vi "LSMcontroller_v64_updatedwaveformhandling.vi"() -> ()   [LabVIEW 2015] (continued)
                                n2114 = property on="downright" class="Bool (strict)"("Value"=w5072) -> ()  [unwired: 2 in, 2 out]
                                }
                                }
                                }
                                }
                                }
                              }
                              n2115 = dll-call lib="phlib.dll" fn="_PH_GetCountRate@8" label="PH_GetCountRate"("devidx"=w5019, "channel"=1) -> (→"Ch1Rate":i32)  [unwired: 5 in, 2 out]
                              n2116 = local read "Stop"() -> (w5021:bool)
                              n2117 = local write "points recorded"(w5018) -> ()
                            }
                          }
                          frame #3 {
                            w5081 = FALSE ("Value (Signaling)")
                            n2118 = call "2pparameters.vi"("command"="get") -> ("params out"=w5075:T10)  [unwired: 1 in]
                            n2119 = Unbundle By Name(w5075) -> ("autoshutter"=w5076:bool)
                            n2120 = case shown="True" w5076 {
                              frame False {
                              }
                              frame True {
                                n2121 = call "shuttercontrol.vi"("command"="close") -> ()  [unwired: 1 in, 1 out]
                              }
                            }
                            n2122 = property on="Start" class="Bool (strict)"("Val(Sgnl)"=w5081) -> ()  [unwired: 2 in, 2 out]
                            n2123 = property on="Start" class="Bool (strict)"("Visible"=TRUE, "DisabledEnum"=T7."Enabled" ("Disabled")) -> ()  [unwired: 2 in, 2 out]
                            n2124 = property on="Stop" class="Bool (strict)"("Val(Sgnl)"=w5081) -> ()  [unwired: 2 in, 2 out]
                            n2125 = property on="Stop" class="Bool (strict)"("Visible"=FALSE, "DisabledEnum"=T7."Disabled" ("Disabled")) -> ()  [unwired: 2 in, 2 out]
                          }
                        }
                      }
                      frame Enabled {
                      }
                    }
                    n2126 = local write "64bit disabled"(TRUE ("64bit disabled")) -> ()
                  }
                }
              }
            }
          }
          event "avpp", "Angle ref", "xpixels ref", "Vx-min ref", "Vx-max ref", "ypixels ref", "Vy-min ref", "Vy-max ref", "ROI Type", "Sampling rate": Value Change {
            n2127 = event-data() -> ()  [unwired: 1 in, 6 out]
            n2128 = local read "avpp"() -> (w5100:i32)
            n2129 = local read "Angle ref"() -> (w5099:dbl)
            n2130 = local read "ROI Type"() -> (w5098:u16)
            n2131 = local read "xpixels ref"() -> (w5095:i32)
            n2132 = local read "Vx-min ref"() -> (w5094:dbl)
            n2133 = local read "Vx-max ref"() -> (w5093:dbl)
            n2134 = local read "ypixels ref"() -> (w5091:i32)
            n2135 = local read "Vy-min ref"() -> (w5092:dbl)
            n2136 = local read "Vy-max ref"() -> (w5088:dbl)
            n2137 = local read "Sampling rate"() -> (w5083:dbl)
            n2138 = local read "# of frames"() -> (w5087:i32)
            n2139 = local read "maxbufferAI"() -> (w5086:i32)
            n2140 = local read "Override AI buffer"() -> (w5084:bool)
            n2141 = call "2pparameters.vi"("command"="get") -> ("params out"=w5097:T10)  [unwired: 1 in]
            n2142 = Bundle By Name(cluster=w5097, "avpp"=w5100, "Angle Img"=w5099, "Xpixels Img"=w5095, "Vx-min Img"=w5094, "VX-max Img"=w5093, "Ypixels Img"=w5091, "Vy-min Img"=w5092, "Vy-max Img"=w5088, "srate"=w5083, "srate Img"=w5083, "measpoints"=w5087, "maxbufferAI"=w5086, "Drawing Mode"=w5098, "Vz-reset"=0.0, "AIoverride"=w5084) -> (w5089:T10)
            n2143 = call "2pparameters.vi"("Params in"=w5089, "command"="set") -> ()  [unwired: 1 out]
          }
          event "# of frames": Value Change {
            n2144 = event-data() -> ()  [unwired: 1 in, 6 out]
            n2145 = local read "Meastab"() -> (w5101:enum32{"X-Y Image", "Linescan", "Timetrace"})
            n2146 = case shown="\"X-Y Image\", Default" w5101 {
              frame "X-Y Image", Default {
                n2147 = local read "# of frames"() -> (w5102:i32)
                n2148 = call "2pparameters.vi"("command"="get") -> ("params out"=w5106:T10)  [unwired: 1 in]
                n2149 = Bundle By Name(cluster=w5106, "measpoints"=w5102) -> (w5103:T10)
                n2150 = call "2pparameters.vi"("Params in"=w5103, "command"="set") -> ()  [unwired: 1 out]
              }
              frame "Linescan" {
                n2151 = local read "srateAODOtt"() -> (w5116:dbl)
                n2152 = local read "# of frames"() -> (w5112:i32)
                n2153 = local read "refreshtime"() -> (w5118:dbl)
                n2154 = local read "bin"() -> (w5113:dbl)
                n2155 = call "tt_timeandsamples.vi"("bin"=w5113, "refreshtime"=w5118, "srateAODOtt"=w5116, "tot#ofsamples"=w5112) -> ("refreshrate"=w5115:dbl, "refreshbuffer"=w5114:i32, "timetracecycles"=w5111:i32)  [unwired: 5 in]
                n2156 = call "2pparameters.vi"("command"="get") -> ("params out"=w5108:T10)  [unwired: 1 in]
                n2157 = Bundle By Name(cluster=w5108, "measpoints"=w5112, "tt_cycles"=w5111, "refreshbuffer"=w5114, "refreshrate"=w5115) -> (w5110:T10)
                n2158 = Reciprocal(x=w5115) -> (1/x=w5117:dbl)
                n2159 = local write "refreshtime"(w5117) -> ()
                n2160 = call "2pparameters.vi"("Params in"=w5110, "command"="set") -> ()  [unwired: 1 out]
              }
              frame "Timetrace" {
                n2161 = local read "srateAODOtt"() -> (w5128:dbl)
                n2162 = local read "# of frames"() -> (w5124:i32)
                n2163 = local read "refreshtime"() -> (w5130:dbl)
                n2164 = local read "bin"() -> (w5125:dbl)
                n2165 = call "tt_timeandsamples.vi"("bin"=w5125, "refreshtime"=w5130, "srateAODOtt"=w5128, "tot#ofsamples"=w5124) -> ("refreshrate"=w5127:dbl, "refreshbuffer"=w5126:i32, "timetracecycles"=w5123:i32)  [unwired: 5 in]
                n2166 = call "2pparameters.vi"("command"="get") -> ("params out"=w5120:T10)  [unwired: 1 in]
                n2167 = Bundle By Name(cluster=w5120, "measpoints"=w5124, "tt_cycles"=w5123, "refreshbuffer"=w5126, "refreshrate"=w5127) -> (w5122:T10)
                n2168 = Reciprocal(x=w5127) -> (1/x=w5129:dbl)
                n2169 = local write "refreshtime"(w5129) -> ()
                n2170 = call "2pparameters.vi"("Params in"=w5122, "command"="set") -> ()  [unwired: 1 out]
              }
            }
          }
          event "srateAODOtt", "refreshtime", "Vx-ref", "Vy-ref", "Vx-min draw", "Vx-max draw", "Vy-min draw", "Vy-max draw", "bin": Value Change {
            n2171 = event-data() -> ()  [unwired: 1 in, 6 out]
            n2172 = local read "ypixels ref"() -> (w5162:i32)
            n2173 = local read "Vy-min draw"() -> (w5138:dbl)
            n2174 = local read "Vy-max draw"() -> (w5137:dbl)
            n2175 = local read "Vx-min draw"() -> (w5140:dbl)
            n2176 = local read "Vx-max draw"() -> (w5139:dbl)
            n2177 = local read "xpixels ref"() -> (w5136:i32)
            n2178 = local read "ROI Type"() -> (w5135:u16)
            n2179 = local read "Pel"() -> (w5134:dbl)
            n2180 = local read "srateAODOtt"() -> (w5144:dbl)
            n2181 = local read "# of frames"() -> (w5149:i32)
            n2182 = local read "refreshtime"() -> (w5142:dbl)
            n2183 = local read "bin"() -> (w5147:dbl)
            n2184 = local read "Override AI buffer"() -> (w5132:bool)
            n2185 = local read "finite samples"() -> (w5156:bool)
            n2186 = local read "srateAODOtt"() -> (w5131:dbl)
            n2187 = local read "srateAODOtt"() -> (w5150:dbl)
            n2188 = local read "continuous"() -> (w5155:bool)
            n2189 = local read "Angle ref"() -> (w5141:dbl)
            n2190 = local read "wavdet"() -> (w5157:bool)
            n2191 = local read "Vx-ref"() -> (w5152:dbl)
            n2192 = local read "Vy-ref"() -> (w5154:dbl)
            n2193 = local read "avpp"() -> (w5153:i32)
            n2194 = call "tt_timeandsamples.vi"("bin"=w5147, "refreshtime"=w5142, "srateAODOtt"=w5144, "tot#ofsamples"=w5149) -> ("refreshrate"=w5145:dbl, "refreshbuffer"=w5146:i32, "timetracecycles"=w5151:i32)  [unwired: 5 in]
            n2195 = local read "bin"() -> (w5148:dbl)
            n2196 = call "2pparameters.vi"("command"="get") -> ("params out"=w5160:T10)  [unwired: 1 in]
            n2197 = Bundle By Name(cluster=w5160, "Drawing Mode"=w5135, "measpoints"=w5149, "tt_cycles"=w5151, "refreshbuffer"=w5146, "refreshrate"=w5145, "Vx-ref"=w5152, "Vy-ref"=w5154, "srate"=w5131, "finite"=w5156, "cont"=w5155, "wavdet"=w5157, "avpp"=w5153, "srateAODO"=w5150, "bufferAI"=w5146, "bin"=w5148, "Angle Img"=w5141, "Vxminref"=w5140, "Vxmaxref"=w5139, "Vyminref"=w5138, "Vymaxref"=w5137, "Xpixels Img"=w5136, "Ypixels Img"=w5162, "Pel"=w5134, "Vz-reset"=0.0, "AIoverride"=w5132) -> (w5158:T10)
            n2198 = Reciprocal(x=w5145) -> (1/x=w5143:dbl)
            n2199 = local write "refreshtime"(w5143) -> ()
            n2200 = call "2pparameters.vi"("Params in"=w5158, "command"="set") -> ()  [unwired: 1 out]
          }
          event "Init": Value Change {
            # "Disabled for conversion to 64 bit"
            n2201 = event-data() -> ()  [unwired: 1 in, 6 out]
            n2202 = disable-structure shown="Disabled" {
              frame Disabled {
                n2203 = flat-sequence {
                  frame #0 {
                    n2204 = local read "Measurement"() -> (w5164:T4)
                    n2205 = case shown="\"Lifetime (scan)\", \"Lifetime (contour)\"" w5164 {
                      frame "X-Y-t movie", Default {
                      }
                      frame "Lifetime (point)" {
                        n2206 = stacked-sequence {
                          frame #0 {
                            n2207 = call "initialize.vi"("mode"=0) -> ()
                          }
                          frame #1 {
                            n2208 = call "calib.vi"() -> ()  [unwired: 1 in]
                          }
                        }
                      }
                      frame "Lifetime (scan)", "Lifetime (contour)" {
                        n2209 = stacked-sequence {
                          frame #0 {
                            n2210 = call "initialize.vi"("mode"=3) -> ()
                          }
                          frame #1 {
                            n2211 = call "calib.vi"() -> ()  [unwired: 1 in]
                          }
                        }
                      }
                    }
                  }
                  frame #1 {
                    n2212 = property on="Start" class="Bool (strict)"("Visible"=TRUE, "DisabledEnum"=T7."Enabled" ("Disabled")) -> ()  [unwired: 2 in, 2 out]
                    n2213 = property on="Init" class="Bool (strict)"("Visible"=FALSE, "DisabledEnum"=T7."Disabled and Grayed Out" ("Disabled"), "Value"=FALSE ("Init")) -> ()  [unwired: 2 in, 2 out]
                  }
                }
              }
              frame Enabled {
              }
            }
            n2214 = local write "64bit disabled"(TRUE ("64bit disabled")) -> ()
          }
          event "Measurement": Value Change {
            n2215 = event-data() -> ()  [unwired: 1 in, 5 out]
            n2216 = case shown="\"X-Y-t movie\"" "Measurement" {
              frame "X-Y-t movie" {
                w5174 = T7."Disabled" ("Disabled")
                w5173 = FALSE ("Visible")
                n2217 = call "2pparameters.vi"("command"="get") -> ("params out"=w5184:T10)  [unwired: 1 in]
                n2218 = local write "graphtab"(T5."image" ("graphtab")) -> ()
                n2219 = local write "Save tab"(enum32{"withsave", "withoutsave"}."withsave" ("Save tab")) -> ()
                n2220 = Bundle By Name(cluster=w5184, "type"="X-Y-t movie") -> (w5182:T10)
                n2221 = call "2pparameters.vi"("Params in"=w5182, "command"="set") -> ()  [unwired: 1 out]
                n2222 = property on="refreshtime" class="DigNum (strict)"("Visible"=FALSE, "DisabledEnum"=T7."Disabled and Grayed Out" ("Disabled")) -> ()  [unwired: 2 in, 2 out]
                n2223 = property on="ttt" class="Enum (strict)"("Visible"=FALSE) -> ()  [unwired: 2 in, 2 out]
                n2224 = property on="# of frames" class="DigNum (strict)"("DisabledEnum"=T7."Enabled" ("Disabled"), "Caption.Text"="# of frames") -> ()  [unwired: 2 in, 2 out]
                n2225 = property on="continuous" class="Bool (strict)"("Visible"=TRUE, "DisabledEnum"=T7."Enabled" ("Disabled")) -> ()  [unwired: 2 in, 2 out]
                n2226 = property on="finite samples" class="Bool (strict)"("Visible"=TRUE, "DisabledEnum"=T7."Enabled" ("Disabled")) -> ()  [unwired: 2 in, 2 out]
                n2227 = property on="avpp" class="DigNum (strict)"("Visible"=TRUE, "DisabledEnum"=T7."Enabled" ("Disabled")) -> ()  [unwired: 2 in, 2 out]
                n2228 = property on="srateAODOtt" class="DigNum (strict)"("Visible"=FALSE, "DisabledEnum"=T7."Disabled" ("Disabled")) -> ()  [unwired: 2 in, 2 out]
                n2229 = local write "save\ndata"(TRUE ("save\ndata")) -> ()
                n2230 = property on="finite samples" class="Bool (strict)"("Val(Sgnl)"=TRUE ("continuous for display")) -> ()  [unwired: 2 in, 2 out]
                n2231 = property on="continuous" class="Bool (strict)"("Value"=FALSE ("continuous for display")) -> ()  [unwired: 2 in, 2 out]
                n2232 = property on="Current Average" class="DigNum (strict)"("Visible"=TRUE, "DisabledEnum"=T7."Enabled" ("Disabled")) -> ()  [unwired: 2 in, 2 out]
                n2233 = property on="img_CH1" class="IntGraph (strict)"("ZScale.Maximum"=7.0 ("Z Scale.Range:Maximum")) -> ()  [unwired: 2 in, 2 out]
                n2234 = property on="Sampling rate" class="DigNum (strict)"("Visible"=TRUE, "DisabledEnum"=T7."Enabled" ("Disabled")) -> ()  [unwired: 2 in, 2 out]
                n2235 = property on="Pel" class="DigNum (strict)"("Visible"=w5173, "DisabledEnum"=w5174) -> ()  [unwired: 2 in, 2 out]
                n2236 = property on="bin" class="DigNum (strict)"("Visible"=w5173, "DisabledEnum"=w5174) -> ()  [unwired: 2 in, 2 out]
                "Meastab" <- enum32{"X-Y Image", "Linescan", "Timetrace"}."X-Y Image" ("Meastab")
                "Zscantab" <- enum32{"withzscan", "withoutzscan", "lifetime"}."withoutzscan" ("Zscantab")
              }
              frame "X-Y-Z stack" {
                w5206 = T7."Disabled" ("Disabled")
                w5205 = FALSE ("Visible")
                n2237 = call "2pparameters.vi"("command"="get") -> ("params out"=w5216:T10)  [unwired: 1 in]
                n2238 = call "2pparameters.vi"("command"="get") -> ("params out"=w5220:T10)  [unwired: 1 in]
                n2239 = Bundle By Name(cluster=w5216, "type"="X-Y-Z stack") -> (w5214:T10)
                n2240 = Unbundle By Name(w5220) -> ("motorref"=w5219:refnum<k7>)
                n2241 = call "2pparameters.vi"("Params in"=w5214, "command"="set") -> ()  [unwired: 1 out]
                n2242 = local write "Zscantab"(enum32{"withzscan", "withoutzscan", "lifetime"}."withzscan" ("Zscantab")) -> ()
                n2243 = local write "Meastab"(enum32{"X-Y Image", "Linescan", "Timetrace"}."X-Y Image" ("Meastab")) -> ()
                n2244 = invoke class="MG17Motor" method="GetPosition"(reference=w5219, "lChanID"=0, "pfPosition"=sgl 0.0) -> ("pfPosition"=w5231:sgl)  [unwired: 2 in, 4 out]
                n2245 = property on="refreshtime" class="DigNum (strict)"("Visible"=FALSE, "DisabledEnum"=T7."Disabled and Grayed Out" ("Disabled")) -> ()  [unwired: 2 in, 2 out]
                n2246 = property on="ttt" class="Enum (strict)"("Visible"=FALSE) -> ()  [unwired: 2 in, 2 out]
                n2247 = Multiply(x=w5231, y=1000.0) -> (x*y=w5230:dbl)
                n2248 = local write "Actual Z position"(w5230) -> ()
                n2249 = local write "Save tab"(enum32{"withsave", "withoutsave"}."withsave" ("Save tab")) -> ()
                n2250 = property on="finite samples" class="Bool (strict)"("Visible"=FALSE, "DisabledEnum"=T7."Disabled and Grayed Out" ("Disabled")) -> ()  [unwired: 2 in, 2 out]
                n2251 = property on="avpp" class="DigNum (strict)"("Visible"=TRUE, "DisabledEnum"=T7."Enabled" ("Disabled")) -> ()  [unwired: 2 in, 2 out]
                n2252 = property on="continuous" class="Bool (strict)"("Visible"=FALSE, "DisabledEnum"=T7."Disabled and Grayed Out" ("Disabled")) -> ()  [unwired: 2 in, 2 out]
                n2253 = property on="img_CH1" class="IntGraph (strict)"("ZScale.Maximum"=7.0 ("Z Scale.Range:Maximum")) -> ()  [unwired: 2 in, 2 out]
                n2254 = property on="srateAODOtt" class="DigNum (strict)"("Visible"=FALSE, "DisabledEnum"=T7."Disabled" ("Disabled")) -> ()  [unwired: 2 in, 2 out]
                n2255 = property on="Pel" class="DigNum (strict)"("Visible"=w5205, "DisabledEnum"=w5206) -> ()  [unwired: 2 in, 2 out]
                n2256 = property on="bin" class="DigNum (strict)"("Visible"=w5205, "DisabledEnum"=w5206) -> ()  [unwired: 2 in, 2 out]
                n2257 = property on="Current Average" class="DigNum (strict)"("Visible"=TRUE, "DisabledEnum"=T7."Enabled" ("Disabled")) -> ()  [unwired: 2 in, 2 out]
                n2258 = property on="# of frames" class="DigNum (strict)"("Caption.Text"="# of slices", "DisabledEnum"=T7."Disabled and Grayed Out" ("Disabled")) -> ()  [unwired: 2 in, 2 out]
                n2259 = local write "save\ndata"(TRUE ("save\ndata")) -> ()
                n2260 = property on="finite samples" class="Bool (strict)"("Val(Sgnl)"=TRUE ("continuous for display")) -> ()  [unwired: 2 in, 2 out]
                n2261 = property on="continuous" class="Bool (strict)"("Value"=FALSE ("continuous for display")) -> ()  [unwired: 2 in, 2 out]
                n2262 = property on="Sampling rate" class="DigNum (strict)"("Visible"=TRUE, "DisabledEnum"=T7."Enabled" ("Disabled")) -> ()  [unwired: 2 in, 2 out]
              }
              frame "X-Y-Z-t movie" {
                w5245 = T7."Disabled" ("Disabled")
                w5244 = FALSE ("Visible")
                n2263 = property on="# of frames" class="DigNum (strict)"("DisabledEnum"=T7."Enabled" ("Disabled")) -> ()  [unwired: 2 in, 2 out]
                n2264 = property on="Current Average" class="DigNum (strict)"("Visible"=TRUE, "DisabledEnum"=T7."Enabled" ("Disabled")) -> ()  [unwired: 2 in, 2 out]
                n2265 = property on="avpp" class="DigNum (strict)"("Visible"=TRUE, "DisabledEnum"=T7."Enabled" ("Disabled")) -> ()  [unwired: 2 in, 2 out]
                n2266 = local write "Save tab"(enum32{"withsave", "withoutsave"}."withsave" ("Save tab")) -> ()
                n2267 = local write "Zscantab"(enum32{"withzscan", "withoutzscan", "lifetime"}."withzscan" ("Zscantab")) -> ()
                n2268 = local write "Meastab"(enum32{"X-Y Image", "Linescan", "Timetrace"}."X-Y Image" ("Meastab")) -> ()
                n2269 = property on="refreshtime" class="DigNum (strict)"("Visible"=FALSE, "DisabledEnum"=T7."Disabled and Grayed Out" ("Disabled")) -> ()  [unwired: 2 in, 2 out]
                n2270 = property on="ttt" class="Enum (strict)"("Visible"=FALSE) -> ()  [unwired: 2 in, 2 out]
                n2271 = call "2pparameters.vi"("command"="get") -> ("params out"=w5255:T10)  [unwired: 1 in]
                n2272 = Bundle By Name(cluster=w5255, "type"="X-Y-Z-t movie") -> (w5253:T10)
                n2273 = property on="continuous" class="Bool (strict)"("Visible"=TRUE, "DisabledEnum"=T7."Enabled" ("Disabled")) -> ()  [unwired: 2 in, 2 out]
                n2274 = property on="finite samples" class="Bool (strict)"("Visible"=TRUE, "DisabledEnum"=T7."Enabled" ("Disabled")) -> ()  [unwired: 2 in, 2 out]
                n2275 = call "2pparameters.vi"("Params in"=w5253, "command"="set") -> ()  [unwired: 1 out]
                n2276 = property on="srateAODOtt" class="DigNum (strict)"("Visible"=FALSE, "DisabledEnum"=T7."Disabled" ("Disabled")) -> ()  [unwired: 2 in, 2 out]
                n2277 = local write "save\ndata"(TRUE ("save\ndata")) -> ()
                n2278 = property on="img_CH1" class="IntGraph (strict)"("ZScale.Maximum"=7.0 ("Z Scale.Range:Maximum")) -> ()  [unwired: 2 in, 2 out]
                n2279 = property on="continuous" class="Bool (strict)"("Value"=FALSE ("continuous for display")) -> ()  [unwired: 2 in, 2 out]
                n2280 = property on="finite samples" class="Bool (strict)"("Value"=TRUE ("continuous for display")) -> ()  [unwired: 2 in, 2 out]
                n2281 = property on="Sampling rate" class="DigNum (strict)"("Visible"=TRUE, "DisabledEnum"=T7."Enabled" ("Disabled")) -> ()  [unwired: 2 in, 2 out]
                n2282 = property on="Pel" class="DigNum (strict)"("Visible"=w5244, "DisabledEnum"=w5245) -> ()  [unwired: 2 in, 2 out]
                n2283 = property on="bin" class="DigNum (strict)"("Visible"=w5244, "DisabledEnum"=w5245) -> ()  [unwired: 2 in, 2 out]
              }
              frame "linescan" {
                w5275 = T7."Enabled" ("Disabled")
                w5274 = TRUE ("Visible")
                w5277 = T7."Enabled" ("Disabled")
                w5276 = TRUE ("Visible")
                n2284 = local write "Meastab"(enum32{"X-Y Image", "Linescan", "Timetrace"}."Linescan" ("Meastab")) -> ()
                n2285 = property on="Current Average" class="DigNum (strict)"("Visible"=TRUE, "DisabledEnum"=T7."Enabled" ("Disabled")) -> ()  [unwired: 2 in, 2 out]
                n2286 = local write "Save tab"(enum32{"withsave", "withoutsave"}."withsave" ("Save tab")) -> ()
                n2287 = local write "Zscantab"(enum32{"withzscan", "withoutzscan", "lifetime"}."withoutzscan" ("Zscantab")) -> ()
                n2288 = property on="refreshtime" class="DigNum (strict)"("Visible"=FALSE, "DisabledEnum"=T7."Disabled and Grayed Out" ("Disabled")) -> ()  [unwired: 2 in, 2 out]
                n2289 = property on="continuous" class="Bool (strict)"("Value"=FALSE ("continuous for display")) -> ()  [unwired: 2 in, 2 out]
                n2290 = property on="finite samples" class="Bool (strict)"("Value"=TRUE ("continuous for display")) -> ()  [unwired: 2 in, 2 out]
                n2291 = property on="ttt" class="Enum (strict)"("Visible"=FALSE) -> ()  [unwired: 2 in, 2 out]
                n2292 = local write "save\ndata"(TRUE ("save\ndata")) -> ()
                n2293 = call "2pparameters.vi"("command"="get") -> ("params out"=w5286:T10)  [unwired: 1 in]
                n2294 = Bundle By Name(cluster=w5286, "type"="linescan") -> (w5284:T10)
                n2295 = property on="# of frames" class="DigNum (strict)"("DisabledEnum"=T7."Enabled" ("Disabled"), "Caption.Text"="# of lines") -> ()  [unwired: 2 in, 2 out]
                n2296 = property on="continuous" class="Bool (strict)"("Visible"=TRUE, "DisabledEnum"=T7."Enabled" ("Disabled")) -> ()  [unwired: 2 in, 2 out]
                n2297 = property on="avpp" class="DigNum (strict)"("Visible"=TRUE, "DisabledEnum"=T7."Enabled" ("Disabled")) -> ()  [unwired: 2 in, 2 out]
                n2298 = property on="finite samples" class="Bool (strict)"("Visible"=TRUE, "DisabledEnum"=T7."Enabled" ("Disabled")) -> ()  [unwired: 2 in, 2 out]
                n2299 = property on="srateAODOtt" class="DigNum (strict)"("Visible"=TRUE, "DisabledEnum"=T7."Enabled" ("Disabled")) -> ()  [unwired: 2 in, 2 out]
                n2300 = call "2pparameters.vi"("Params in"=w5284, "command"="set") -> ()  [unwired: 1 out]
                n2301 = property on="Pel" class="DigNum (strict)"("Visible"=w5276, "DisabledEnum"=w5277) -> ()  [unwired: 2 in, 2 out]
                n2302 = property on="bin" class="DigNum (strict)"("Visible"=w5276, "DisabledEnum"=w5277) -> ()  [unwired: 2 in, 2 out]
                n2303 = property on="Sampling rate" class="DigNum (strict)"("Visible"=FALSE, "DisabledEnum"=T7."Disabled" ("Disabled")) -> ()  [unwired: 2 in, 2 out]
                n2304 = property on="Pel" class="DigNum (strict)"("Visible"=w5274, "DisabledEnum"=w5275) -> ()  [unwired: 2 in, 2 out]
                n2305 = property on="bin" class="DigNum (strict)"("Visible"=w5274, "DisabledEnum"=w5275) -> ()  [unwired: 2 in, 2 out]
              }
              frame "Timetrace" {
                w5307 = T7."Enabled" ("Disabled")
                w5306 = TRUE ("Visible")
                n2306 = call "2pparameters.vi"("command"="get") -> ("params out"=w5312:T10)  [unwired: 1 in]
                n2307 = local write "Meastab"(enum32{"X-Y Image", "Linescan", "Timetrace"}."Timetrace" ("Meastab")) -> ()
                n2308 = Unbundle By Name(w5312) -> ("Angle draw"=w5314:dbl)
                n2309 = local write "Zscantab"(enum32{"withzscan", "withoutzscan", "lifetime"}."withoutzscan" ("Zscantab")) -> ()
                n2310 = property on="# of frames" class="DigNum (strict)"("DisabledEnum"=T7."Enabled" ("Disabled"), "Caption.Text"="# of samples") -> ()  [unwired: 2 in, 2 out]
                n2311 = property on="refreshtime" class="DigNum (strict)"("Visible"=TRUE, "DisabledEnum"=T7."Enabled" ("Disabled")) -> ()  [unwired: 2 in, 2 out]
                n2312 = property on="avpp" class="DigNum (strict)"("Visible"=FALSE, "DisabledEnum"=T7."Disabled and Grayed Out" ("Disabled")) -> ()  [unwired: 2 in, 2 out]
                n2313 = property on="Current Average" class="DigNum (strict)"("Visible"=FALSE, "DisabledEnum"=T7."Disabled and Grayed Out" ("Disabled")) -> ()  [unwired: 2 in, 2 out]
                n2314 = local write "Angle drawing"(w5314) -> ()
                n2315 = property on="ttt" class="Enum (strict)"("Visible"=TRUE) -> ()  [unwired: 2 in, 2 out]
                n2316 = property on="continuous" class="Bool (strict)"("Visible"=TRUE, "DisabledEnum"=T7."Enabled" ("Disabled")) -> ()  [unwired: 2 in, 2 out]
                n2317 = property on="finite samples" class="Bool (strict)"("Visible"=TRUE, "DisabledEnum"=T7."Enabled" ("Disabled")) -> ()  [unwired: 2 in, 2 out]
                n2318 = local write "save\ndata"(TRUE ("save\ndata")) -> ()
                n2319 = property on="finite samples" class="Bool (strict)"("Val(Sgnl)"=TRUE ("continuous for display")) -> ()  [unwired: 2 in, 2 out]
                n2320 = property on="continuous" class="Bool (strict)"("Value"=FALSE ("continuous for display")) -> ()  [unwired: 2 in, 2 out]
                n2321 = local write "Save tab"(enum32{"withsave", "withoutsave"}."withsave" ("Save tab")) -> ()
                n2322 = property on="srateAODOtt" class="DigNum (strict)"("Visible"=TRUE, "DisabledEnum"=T7."Enabled" ("Disabled")) -> ()  [unwired: 2 in, 2 out]
                n2323 = call "2pparameters.vi"("command"="get") -> ("params out"=w5319:T10)  [unwired: 1 in]
                n2324 = Bundle By Name(cluster=w5319, "type"="Timetrace") -> (w5317:T10)
                n2325 = property on="Sampling rate" class="DigNum (strict)"("Visible"=FALSE, "DisabledEnum"=T7."Disabled" ("Disabled")) -> ()  [unwired: 2 in, 2 out]
                n2326 = property on="Pel" class="DigNum (strict)"("Visible"=w5306, "DisabledEnum"=w5307) -> ()  [unwired: 2 in, 2 out]
                n2327 = property on="bin" class="DigNum (strict)"("Visible"=w5306, "DisabledEnum"=w5307) -> ()  [unwired: 2 in, 2 out]
                n2328 = call "2pparameters.vi"("Params in"=w5317, "command"="set") -> ()  [unwired: 1 out]
              }
              frame "Lifetime (point)" {
                w5340 = T7."Enabled" ("Disabled")
                w5339 = TRUE ("Visible")
                n2329 = property on="Pel" class="DigNum (strict)"("Visible"=w5339, "DisabledEnum"=w5340) -> ()  [unwired: 2 in, 2 out]
                n2330 = property on="bin" class="DigNum (strict)"("Visible"=w5339, "DisabledEnum"=w5340) -> ()  [unwired: 2 in, 2 out]
                n2331 = property on="ttt" class="Enum (strict)"("Visible"=FALSE) -> ()  [unwired: 2 in, 2 out]
                n2332 = local write "Zscantab"(enum32{"withzscan", "withoutzscan", "lifetime"}."lifetime" ("Zscantab")) -> ()
                n2333 = local write "graphtab"(T5."Lifetime" ("graphtab")) -> ()
                n2334 = local write "Meastab"(enum32{"X-Y Image", "Linescan", "Timetrace"}."Timetrace" ("Meastab")) -> ()
                n2335 = call "lifetimeparameters.vi"("command"="get") -> ("Params out"=w5347:T19)  [unwired: 1 in]
                n2336 = Unbundle By Name(w5347) -> ("initialized"=w5348:bool)
                n2337 = property on="srateAODOtt" class="DigNum (strict)"("Visible"=TRUE, "DisabledEnum"=T7."Enabled" ("Disabled")) -> ()  [unwired: 2 in, 2 out]
                n2338 = case shown="False" w5348 {
                  frame False {
                    n2339 = property on="Init" class="Bool (strict)"("Visible"=TRUE, "DisabledEnum"=T7."Enabled" ("Disabled")) -> ()  [unwired: 2 in, 2 out]
                    n2340 = property on="Start" class="Bool (strict)"("Visible"=FALSE, "DisabledEnum"=T7."Disabled and Grayed Out" ("Disabled")) -> ()  [unwired: 2 in, 2 out]
                  }
                  frame True {
                  }
                }
                n2341 = property on="Sampling rate" class="DigNum (strict)"("Visible"=FALSE, "DisabledEnum"=T7."Disabled" ("Disabled")) -> ()  [unwired: 2 in, 2 out]
              }
              frame "Lifetime (scan)" {
                w5357 = T7."Disabled" ("Disabled")
                w5356 = FALSE ("Visible")
                n2342 = call "lifetimeparameters.vi"("command"="get") -> ("Params out"=w5369:T19)  [unwired: 1 in]
                n2343 = local write "graphtab"(T5."image" ("graphtab")) -> ()
                n2344 = local write "Save tab"(enum32{"withsave", "withoutsave"}."withsave" ("Save tab")) -> ()
                n2345 = local write "Meastab"(enum32{"X-Y Image", "Linescan", "Timetrace"}."X-Y Image" ("Meastab")) -> ()
                n2346 = local write "Zscantab"(enum32{"withzscan", "withoutzscan", "lifetime"}."lifetime" ("Zscantab")) -> ()
                n2347 = Unbundle By Name(w5369) -> ("initialized"=w5368:bool)
                n2348 = property on="ttt" class="Enum (strict)"("Visible"=FALSE) -> ()  [unwired: 2 in, 2 out]
                n2349 = property on="refreshtime" class="DigNum (strict)"("Visible"=FALSE, "DisabledEnum"=T7."Disabled and Grayed Out" ("Disabled")) -> ()  [unwired: 2 in, 2 out]
                n2350 = property on="Pel" class="DigNum (strict)"("Visible"=w5356, "DisabledEnum"=w5357) -> ()  [unwired: 2 in, 2 out]
                n2351 = property on="bin" class="DigNum (strict)"("Visible"=w5356, "DisabledEnum"=w5357) -> ()  [unwired: 2 in, 2 out]
                n2352 = property on="save data" class="Bool (strict)"("Visible"=TRUE, "DisabledEnum"=T7."Enabled" ("Disabled"), "Value"=TRUE ("Visible")) -> ()  [unwired: 2 in, 2 out]
                n2353 = case shown="False" w5368 {
                  frame False {
                    n2354 = property on="Init" class="Bool (strict)"("Visible"=TRUE, "DisabledEnum"=T7."Enabled" ("Disabled")) -> ()  [unwired: 2 in, 2 out]
                    n2355 = property on="Start" class="Bool (strict)"("Visible"=FALSE, "DisabledEnum"=T7."Disabled and Grayed Out" ("Disabled")) -> ()  [unwired: 2 in, 2 out]
                  }
                  frame True {
                  }
                }
                n2356 = call "2pparameters.vi"("command"="get") -> ("params out"=w5374:T10)  [unwired: 1 in]
                n2357 = property on="continuous" class="Bool (strict)"("Visible"=TRUE, "DisabledEnum"=T7."Disabled and Grayed Out" ("Disabled")) -> ()  [unwired: 2 in, 2 out]
                n2358 = property on="finite samples" class="Bool (strict)"("Visible"=TRUE, "DisabledEnum"=T7."Enabled" ("Disabled")) -> ()  [unwired: 2 in, 2 out]
                n2359 = Bundle By Name(cluster=w5374, "type"="Lifetime (scan)") -> (w5372:T10)
                n2360 = call "2pparameters.vi"("Params in"=w5372, "command"="set") -> ()  [unwired: 1 out]
                n2361 = property on="finite samples" class="Bool (strict)"("Val(Sgnl)"=TRUE ("continuous for display")) -> ()  [unwired: 2 in, 2 out]
                n2362 = property on="continuous" class="Bool (strict)"("Value"=FALSE ("continuous for display")) -> ()  [unwired: 2 in, 2 out]
                n2363 = property on="srateAODOtt" class="DigNum (strict)"("Visible"=FALSE, "DisabledEnum"=T7."Disabled" ("Disabled")) -> ()  [unwired: 2 in, 2 out]
                n2364 = property on="# of frames" class="DigNum (strict)"("DisabledEnum"=T7."Enabled" ("Disabled"), "Caption.Text"="# of frames") -> ()  [unwired: 2 in, 2 out]
                n2365 = property on="img_CH1" class="IntGraph (strict)"("ZScale.Maximum"=12.5 ("Z Scale.Range:Maximum")) -> ()  [unwired: 2 in, 2 out]
                n2366 = property on="Current Average" class="DigNum (strict)"("Visible"=TRUE, "DisabledEnum"=T7."Enabled" ("Disabled")) -> ()  [unwired: 2 in, 2 out]
                n2367 = property on="Sampling rate" class="DigNum (strict)"("Visible"=TRUE, "DisabledEnum"=T7."Enabled" ("Disabled")) -> ()  [unwired: 2 in, 2 out]
                n2368 = property on="avpp" class="DigNum (strict)"("Visible"=TRUE, "DisabledEnum"=T7."Enabled" ("Disabled")) -> ()  [unwired: 2 in, 2 out]
              }
              frame "Lifetime (contour)" {
                w5398 = T7."Enabled" ("Disabled")
                w5397 = TRUE ("Visible")
                n2369 = call "2pparameters.vi"("command"="get") -> ("params out"=w5405:T10)  [unwired: 1 in]
                n2370 = property on="# of frames" class="DigNum (strict)"("DisabledEnum"=T7."Enabled" ("Disabled"), "Caption.Text"="# of samples") -> ()  [unwired: 2 in, 2 out]
                n2371 = property on="refreshtime" class="DigNum (strict)"("Visible"=TRUE, "DisabledEnum"=T7."Enabled" ("Disabled")) -> ()  [unwired: 2 in, 2 out]
                n2372 = Unbundle By Name(w5405) -> ("Angle draw"=w5407:dbl)
                n2373 = property on="avpp" class="DigNum (strict)"("Visible"=FALSE, "DisabledEnum"=T7."Disabled and Grayed Out" ("Disabled")) -> ()  [unwired: 2 in, 2 out]
                n2374 = property on="Current Average" class="DigNum (strict)"("Visible"=FALSE, "DisabledEnum"=T7."Disabled and Grayed Out" ("Disabled")) -> ()  [unwired: 2 in, 2 out]
                n2375 = local write "Angle drawing"(w5407) -> ()
                n2376 = local write "Save tab"(enum32{"withsave", "withoutsave"}."withsave" ("Save tab")) -> ()
                n2377 = local write "Zscantab"(enum32{"withzscan", "withoutzscan", "lifetime"}."lifetime" ("Zscantab")) -> ()
                n2378 = local write "graphtab"(T5."Lifetime" ("graphtab")) -> ()
                n2379 = local write "Meastab"(enum32{"X-Y Image", "Linescan", "Timetrace"}."Timetrace" ("Meastab")) -> ()
                n2380 = property on="ttt" class="Enum (strict)"("Visible"=TRUE) -> ()  [unwired: 2 in, 2 out]
                n2381 = call "lifetimeparameters.vi"("command"="get") -> ("Params out"=w5429:T19)  [unwired: 1 in]
                n2382 = property on="finite samples" class="Bool (strict)"("Val(Sgnl)"=TRUE ("continuous for display")) -> ()  [unwired: 2 in, 2 out]
                n2383 = local write "save\ndata"(TRUE ("save\ndata")) -> ()
                n2384 = Unbundle By Name(w5429) -> ("initialized"=w5430:bool)
                n2385 = property on="continuous" class="Bool (strict)"("Visible"=TRUE, "DisabledEnum"=T7."Enabled" ("Disabled")) -> ()  [unwired: 2 in, 2 out]
                n2386 = property on="finite samples" class="Bool (strict)"("Visible"=TRUE, "DisabledEnum"=T7."Enabled" ("Disabled")) -> ()  [unwired: 2 in, 2 out]
                n2387 = property on="Pel" class="DigNum (strict)"("Visible"=w5397, "DisabledEnum"=w5398) -> ()  [unwired: 2 in, 2 out]
                n2388 = property on="bin" class="DigNum (strict)"("Visible"=w5397, "DisabledEnum"=w5398) -> ()  [unwired: 2 in, 2 out]
                n2389 = property on="continuous" class="Bool (strict)"("Value"=FALSE ("continuous for display")) -> ()  [unwired: 2 in, 2 out]
                n2390 = case shown="False" w5430 {
                  frame False {
                    n2391 = property on="Init" class="Bool (strict)"("Visible"=TRUE, "DisabledEnum"=T7."Enabled" ("Disabled")) -> ()  [unwired: 2 in, 2 out]
                    n2392 = property on="Start" class="Bool (strict)"("Visible"=FALSE, "DisabledEnum"=T7."Disabled and Grayed Out" ("Disabled")) -> ()  [unwired: 2 in, 2 out]
                  }
                  frame True {
                  }
                }
                n2393 = property on="srateAODOtt" class="DigNum (strict)"("Visible"=TRUE, "DisabledEnum"=T7."Enabled" ("Disabled")) -> ()  [unwired: 2 in, 2 out]
                n2394 = call "2pparameters.vi"("command"="get") -> ("params out"=w5409:T10)  [unwired: 1 in]
                n2395 = Bundle By Name(cluster=w5409, "type"="Timetrace") -> (w5403:T10)
                n2396 = call "2pparameters.vi"("Params in"=w5403, "command"="set") -> ()  [unwired: 1 out]
                n2397 = property on="Sampling rate" class="DigNum (strict)"("Visible"=FALSE, "DisabledEnum"=T7."Disabled" ("Disabled")) -> ()  [unwired: 2 in, 2 out]
              }
            }
          }
          event "Laserpower \n(%)": Value Change {
            n2398 = event-data() -> ("OldVal"=w5438:dbl, "NewVal"=w5439:dbl)  [unwired: 1 in, 4 out]
            n2399 = Not Equal?(x=w5438, y=w5439) -> (x != y?=w5440:bool)
            n2400 = case shown="True" w5440 {
              tunnel: w5439 -> [_ w5442]
              frame False {
              }
              frame True {
                n2401 = local read "wavelength(nm)"() -> (w5443:dbl)
                n2402 = call "configuration.vi"("command"="get") -> ("config out"=w5447:T11)  [unwired: 2 in, 1 out]
                n2403 = call "pockelscellcalibration.vi"("l"=w5443, "T"=w5442) -> ("Vout"=w5441:dbl)
                n2404 = Unbundle By Name(w5447) -> ("Vto2P"=w5446:i32, "AOlines"=w5445:tag[])
                n2405 = property on="lpow" class="DigNum (strict)"("Value"=w5442) -> ()  [unwired: 2 in, 2 out]
                n2406 = local write "Vpockels"(w5441) -> ()
                n2407 = Index Array(array=w5445, index=w5446) -> (element=w5444:tag)
                n2408 = call-poly <vilib>:"DAQmx Create Virtual Channel.vi"("physical channels"=w5444) -> ("task out"=w5450:refnum<k21>, "error out"=w5449:errorcluster)  [unwired: 13 in]
                n2409 = call-poly <vilib>:"DAQmx Write.vi"("task/channels in"=w5450, "data"=w5441, "error in"=w5449) -> ("task out"=w5451:refnum<k21>, "error out"=w5452:errorcluster)  [unwired: 10 in, 1 out]
                n2410 = call <vilib>:"DAQmx Start Task.vi"("task/channels in"=w5451, "error in"=w5452) -> ("task out"=w5453:refnum<k21>, "error out"=w5454:errorcluster)  [unwired: 12 in]
                n2411 = call <vilib>:"DAQmx Stop Task.vi"("task/channels in"=w5453, "error in"=w5454) -> ("task out"=w5455:refnum<k21>, "error out"=w5456:errorcluster)  [unwired: 12 in]
                n2412 = call <vilib>:"DAQmx Clear Task.vi"("task in"=w5455, "error in"=w5456) -> ()  [unwired: 13 in, 1 out]
              }
            }
          }
          event "lpow": Value Change {
            n2413 = event-data() -> ("OldVal"=w5457:dbl, "NewVal"=w5458:dbl)  [unwired: 1 in, 4 out]
            n2414 = Not Equal?(x=w5457, y=w5458) -> (x != y?=w5459:bool)
            n2415 = case shown="True" w5459 {
              tunnel: w5458 -> [_ w5462]
              frame False {
              }
              frame True {
                n2416 = local read "wavelength(nm)"() -> (w5461:dbl)
                n2417 = call "pockelscellcalibration.vi"("l"=w5461, "T"=w5462) -> ("Vout"=w5460:dbl)
                n2418 = call "configuration.vi"("command"="get") -> ("config out"=w5466:T11)  [unwired: 2 in, 1 out]
                n2419 = Unbundle By Name(w5466) -> ("Vto2P"=w5465:i32, "AOlines"=w5464:tag[])
                n2420 = local write "Vpockels"(w5460) -> ()
                n2421 = property on="Laserpower \n(%)" class="Slide (strict)"("Value"=w5462) -> ()  [unwired: 2 in, 2 out]
                n2422 = Index Array(array=w5464, index=w5465) -> (element=w5463:tag)
                n2423 = call-poly <vilib>:"DAQmx Create Virtual Channel.vi"("physical channels"=w5463) -> ("task out"=w5469:refnum<k21>, "error out"=w5468:errorcluster)  [unwired: 13 in]
                n2424 = call-poly <vilib>:"DAQmx Write.vi"("task/channels in"=w5469, "data"=w5460, "error in"=w5468) -> ("task out"=w5470:refnum<k21>, "error out"=w5471:errorcluster)  [unwired: 10 in, 1 out]
                n2425 = call <vilib>:"DAQmx Start Task.vi"("task/channels in"=w5470, "error in"=w5471) -> ("task out"=w5472:refnum<k21>, "error out"=w5473:errorcluster)  [unwired: 12 in]
                n2426 = call <vilib>:"DAQmx Stop Task.vi"("task/channels in"=w5472, "error in"=w5473) -> ("task out"=w5474:refnum<k21>, "error out"=w5475:errorcluster)  [unwired: 12 in]
                n2427 = call <vilib>:"DAQmx Clear Task.vi"("task in"=w5474, "error in"=w5475) -> ()  [unwired: 13 in, 1 out]
              }
            }
          }
          event "sealtest": Value Change {
            n2428 = event-data() -> ()  [unwired: 1 in, 6 out]
            n2429 = case shown="True" "sealtest" {
              frame False {
              }
              frame True {
                n2430 = stacked-sequence {
                  seq-local: [w5477 _ _ _ _ _] -> [_ w5510 _ w5562 _ _]
                  frame #0 {
                    n2431 = stacked-sequence {
                      tunnel: [_ w5489 _] -> w5477
                      frame #0 {
                        n2432 = call "2pparameters.vi"("command"="get") -> ("params out"=w5482:T10)  [unwired: 1 in]
                        n2433 = Unbundle By Name(w5482) -> ("autoshutter"=w5483:bool)
                        n2434 = local read "OCchecked?"() -> (w5480:bool)
                        n2435 = call "sealtestwfparams.vi"("command"="set") -> ()  [unwired: 6 in, 1 out]
                        n2436 = case shown="False" w5480 {
                          frame False {
                            n2437 = One Button Dialog(message="Is the OC gain correct?", button name ("OK")="ok") -> (true=w5484:bool)
                            n2438 = local write "OCchecked?"(w5484) -> ()
                          }
                          frame True {
                          }
                        }
                        n2439 = case shown="True" w5483 {
                          frame False {
                          }
                          frame True {
                            n2440 = call "shuttercontrol.vi"("command"="close") -> ()  [unwired: 1 in, 1 out]
                          }
                        }
                        n2441 = call "allAI-temp.vi"("command"=enum16{"get", "set", "clear", "append"}."clear") -> ()  [unwired: 3 in, 2 out]
                      }
                      frame #1 {
                        n2442 = call "sealtestwfparams.vi"("command"="get") -> ("Params out"=w5495:T22)  [unwired: 6 in]
                        n2443 = Unbundle By Name(w5495) -> ("AO parameters"=w5493:T23)
                        n2444 = Index Array(array=w5493, index=0) -> (element=w5492:T24)
                        n2445 = call "generateRampedSquareWave_fromAOparameters.vi"("AO params"=w5492) -> ("Waveform"=w5488:waveform(dbl), "wflength"=w5489:i32)
                        n2446 = Build Array(w5488) -> (w5491:waveform(dbl)[])
                        n2447 = call "waveformssealtestbuffer.vi"("AO wf in"=w5491, "command"="set") -> ()  [unwired: 1 out]
                      }
                      frame #2 {
                        n2448 = local read "Vholding (mV)"() -> (w5498:sgl)
                        n2449 = local read "Current Clamp"() -> (w5504:bool)
                        n2450 = local read "Voltage Clamp"() -> (w5503:bool)
                        n2451 = local read "OCgain"() -> (w5499:sgl)
                        n2452 = local read "CC_ICgain"() -> (w5502:dbl)
                        n2453 = local read "holdon"() -> (w5497:bool)
                        n2454 = call "patchparameters.vi"("command"="get") -> ("Params out"=w5506:T13)  [unwired: 1 in]
                        n2455 = Bundle By Name(cluster=w5506, "VC"=w5503, "CC"=w5504, "CC_icg (pA/mv)"=w5502, "VC_icg (mV/mV)"=10.0, "OCG (mV/pA)"=w5499, "OVG (mV/mV)"=0.1, "Vhold (mV)"=w5498, "holdon"=w5497) -> (w5505:T13)
                        n2456 = call "patchparameters.vi"("Params in"=w5505, "command"="set") -> ()  [unwired: 1 out]
                      }
                    }
                  }
                  frame #1 {
                    w5509 = 2
                    n2457 = call "patchparameters.vi"("command"="get") -> ("Params out"=w5517:T13)  [unwired: 1 in]
                    n2458 = Unbundle By Name(w5517) -> ("holdon"=w5516:bool, "Vhold (mV)"=w5515:sgl, "CC_icg (pA/mv)"=w5523:sgl, "CC"=w5521:bool, "VC_icg (mV/mV)"=w5522:sgl)
                    n2459 = Select(t=w5523, s=w5521, f=w5522) -> (s? t:f=w5524:sgl)
                    n2460 = To Single Precision Float(number=0.001 ("y")) -> (single precision float=w5525:sgl)
                    n2461 = Compound Arithmetic op=MULTIPLY(w5515, w5524, w5525) -> (w5519:sgl)
                    n2462 = case shown="False" w5516 {
                      tunnel: w5519 -> [_ w5537]
                      tunnel: [0.0 w5537] -> w5512
                      frame False {
                      }
                      frame True {
                      }
                    }
                    n2463 = Greater Than 0?(x=w5509) -> (x > 0?=w5511:bool)
                    n2464 = case shown="True" w5511 {
                      tunnel: w5510 -> [_ w5526]
                      tunnel: w5509 -> [_ w5529]
                      frame False {
                      }
                      frame True {
                        n2465 = Initialize Array(sgl 0.0 ("element"), w5529, w5526) -> (w5527:sgl[][])
                        n2466 = call "allAI-temp.vi"("array in"=w5527, "command"=enum16{"get", "set", "clear", "append"}."set") -> ()  [unwired: 2 in, 2 out]
                      }
                    }
                    n2467 = flat-sequence {
                      tunnel: w5510 -> [w5533]
                      tunnel: w5510 -> [w5532]
                      tunnel: [w5532] -> w5514
                      tunnel: [w5531] -> w5513
                      tunnel: w5512 -> [w5531]
                      tunnel: w5514 -> [w5535]
                      tunnel: w5513 -> [w5534]
                      frame #0 {
                        n2468 = call "prepAI_sealtest.vi"("samples per channel"=w5533) -> ()  [unwired: 2 in]
                      }
                      frame #1 {
                        n2469 = call "prepAO_sealtest.vi"("Vhold"=w5534, "samples per channel"=w5535) -> ()  [unwired: 1 in]
                      }
                    }
                  }
                  frame #2 {
                    n2470 = stacked-sequence {
                      frame #0 {
                        n2471 = call "tempconfigAO.vi"("command"="get") -> ("Temp Config out"=w5541:T25)  [unwired: 1 in]
                        n2472 = Unbundle By Name(w5541) -> ("AO"=w5542:refnum<k21>[], "E_AO"=w5543:errorcluster[])
                        n2473 = for {
                          tunnel: w5542 -> [w5551] mode=indexing
                          tunnel: w5543 -> [w5550] mode=indexing
                          tunnel: [w5549] -> w5545 mode=indexing
                          tunnel: [w5548] -> w5546 mode=indexing
                          n2474 = call <vilib>:"DAQmx Start Task.vi"("task/channels in"=w5551, "error in"=w5550) -> ("task out"=w5549:refnum<k21>, "error out"=w5548:errorcluster)  [unwired: 12 in]
                        }
                        n2475 = call "tempconfigAO.vi"("command"="get") -> ("Temp Config out"=w5544:T25)  [unwired: 1 in]
                        n2476 = Bundle By Name(cluster=w5544, "AO"=w5545, "E_AO"=w5546) -> (w5547:T25)
                        n2477 = call "tempconfigAO.vi"("Temp Config in"=w5547, "command"="set") -> ()  [unwired: 1 out]
                      }
                      frame #1 {
                        n2478 = call "tempconfigAI.vi"("command"="get") -> ("Temp Config out"=w5553:T26)  [unwired: 1 in]
                        n2479 = Unbundle By Name(w5553) -> ("AI"=w5558:refnum<k21>, "E_AI"=w5559:errorcluster)
                        n2480 = call <vilib>:"DAQmx Start Task.vi"("task/channels in"=w5558, "error in"=w5559) -> ("task out"=w5560:refnum<k21>, "error out"=w5561:errorcluster)  [unwired: 12 in]
                        n2481 = call "tempconfigAI.vi"("command"="get") -> ("Temp Config out"=w5555:T26)  [unwired: 1 in]
                        n2482 = Bundle By Name(cluster=w5555, "AI"=w5560, "E_AI"=w5561) -> (w5557:T26)
                        n2483 = call "tempconfigAI.vi"("Temp Config in"=w5557, "command"="set") -> ()  [unwired: 1 out]
                      }
                    }
                  }
                  frame #3 {
                    n2484 = while {
                      tunnel: w5562 -> [w5563]
                      stop <- w5564 stop-if-true
                      n2485 = local read "sealtest"() -> (w5567:bool)
                      n2486 = Not(x=w5567) -> (.not. x?=w5566:bool)
                      n2487 = case shown="False" w5566 {
                        tunnel: w5563 -> [w5568 _]
                        frame False {
                          n2488 = stacked-sequence {
                            seq-local: [_ _ _ w5607 _ _] -> [_ _ _ _ w5663 _]
                            seq-local: [w5569 _ _ _ _ _] -> [_ w5578 _ w5600 w5652 w5683]
                            tunnel: w5568 -> [_ _ w5586 _ w5651 _]
                            frame #0 {
                              n2489 = call "patchparameters.vi"("command"="get") -> ("Params out"=w5576:T13)  [unwired: 1 in]
                              n2490 = local read "Vholding (mV)"() -> (w5573:sgl)
                              n2491 = Unbundle By Name(w5576) -> ("Vhold (mV)"=w5572:sgl, "holdon"=w5575:bool)
                              n2492 = local read "holdon"() -> (w5574:bool)
                              n2493 = Not Equal?(x=w5573, y=w5572) -> (x != y?=w5571:bool)
                              n2494 = Not Equal?(x=w5575, y=w5574) -> (x != y?=w5570:bool)
                              n2495 = Or(x=w5571, y=w5570) -> (x .or. y?=w5569:bool)
                            }
                            frame #1 {
                              n2496 = case shown="True" w5578 {
                                frame False {
                                }
                                frame True {
                                n2497 = local read "Vholding (mV)"() -> (w5581:sgl)
                                n2498 = local read "holdon"() -> (w5579:bool)
                                n2499 = call "patchparameters.vi"("command"="get") -> ("Params out"=w5582:T13)  [unwired: 1 in]
                                n2500 = Bundle By Name(cluster=w5582, "Vhold (mV)"=w5581, "holdon"=w5579) -> (w5580:T13)
                                n2501 = call "patchparameters.vi"("Params in"=w5580, "command"="set") -> ()  [unwired: 1 out]
                                }
                              }
                            }
                            frame #2 {
                              n2502 = call "tempconfigAI.vi"("command"="get") -> ("Temp Config out"=w5596:T26)  [unwired: 1 in]
                              n2503 = Unbundle By Name(w5596) -> ("AI"=w5595:refnum<k21>, "E_AI"=w5594:errorcluster)
                              n2504 = call-poly <vilib>:"DAQmx Read.vi"("task/channels in"=w5595, "number of samples per channel"=w5586, "timeout"=10.0, "error in"=w5594) -> ("task out"=w5590:refnum<k21>, "data"=w5587:i16[][], "error out"=w5599:errorcluster)  [unwired: 9 in]
                              n2505 = call "tempconfigAI.vi"("command"="get") -> ("Temp Config out"=w5591:T26)  [unwired: 1 in]
                              n2506 = Bundle By Name(cluster=w5591, "AI"=w5590, "E_AI"=w5599) -> (w5598:T26)
                              n2507 = To Single Precision Float(number=w5587) -> (single precision float=w5589:sgl[][])
                              n2508 = call "tempconfigAI.vi"("Temp Config in"=w5598, "command"="set") -> ()  [unwired: 1 out]
                              n2509 = call "allAI-temp.vi"("array in"=w5589, "command"=enum16{"get", "set", "clear", "append"}."set") -> ()  [unwired: 2 in, 2 out]
                            }
                            frame #3 {
                              n2510 = case shown="True" w5600 {
                                frame False {
                                }
                                frame True {
                                n2511 = call "tempconfigAO.vi"("command"="get") -> ("Temp Config out"=w5640:T25)  [unwired: 1 in]
                                n2512 = Unbundle By Name(w5640) -> ("AO"=w5639:refnum<k21>[], "E_AO"=w5638:errorcluster[])
                                n2513 = call "tempconfigAI.vi"("command"="get") -> ("Temp Config out"=w5627:T26)  [unwired: 1 in]
                                n2514 = Unbundle By Name(w5627) -> ("AI"=w5628:refnum<k21>, "E_AI"=w5629:errorcluster)
                                n2515 = for {
                                tunnel: w5639 -> [w5644] mode=indexing
                                tunnel: w5638 -> [w5643] mode=indexing
                                tunnel: [w5642] -> w5634 mode=indexing
                                n2516 = call <vilib>:"DAQmx Stop Task.vi"("task/channels in"=w5644, "error in"=w5643) -> ("task out"=w5645:refnum<k21>, "error out"=w5646:errorcluster)  [unwired: 12 in]
                                n2517 = call <vilib>:"DAQmx Clear Task.vi"("task in"=w5645, "error in"=w5646) -> ("error out"=w5642:errorcluster)  [unwired: 13 in]
                                }
                                n2518 = call <vilib>:"DAQmx Stop Task.vi"("task/channels in"=w5628, "error in"=w5629) -> ("task out"=w5625:refnum<k21>, "error out"=w5624:errorcluster)  [unwired: 12 in]
                                n2519 = call <vilib>:"DAQmx Clear Task.vi"("task in"=w5625, "error in"=w5624) -> ("error out"=w5623:errorcluster)  [unwired: 13 in]
                                n2520 = call "tempconfigAO.vi"("command"="get") -> ("Temp Config out"=w5635:T25)  [unwired: 1 in]
                                n2521 = Bundle By Name(cluster=w5635, "E_AO"=w5634) -> (w5633:T25)
                                n2522 = call "tempconfigAI.vi"("command"="get") -> ("Temp Config out"=w5631:T26)  [unwired: 1 in]
                                n2523 = Bundle By Name(cluster=w5631, "E_AI"=w5623) -> (w5622:T26)
                                n2524 = call "tempconfigAO.vi"("Temp Config in"=w5633, "command"="set") -> ()  [unwired: 1 out]
                                n2525 = call "tempconfigAI.vi"("Temp Config in"=w5622, "command"="set") -> ()  [unwired: 1 out]
                                }
                              }
                              n2526 = call "allAI-temp.vi"("command"=enum16{"get", "set", "clear", "append"}."get") -> ("array out"=w5604:sgl[][])  [unwired: 3 in, 1 out]
                              n2527 = call "tempconfigAI.vi"("command"="get") -> ("Temp Config out"=w5617:T26)  [unwired: 1 in]
                              n2528 = call "tempconfigAI.vi"("command"="get") -> ("Temp Config out"=w5619:T26)  [unwired: 1 in]
                              n2529 = Unbundle By Name(w5617) -> ("header"=w5615:dbl[])
                              n2530 = Unbundle By Name(w5619) -> ("header"=w5621:dbl[])
                              n2531 = Index Array(array=w5604, index (row) #1=1 ("index (row)"), index (row) #2=0 ("index (row)")) -> (element #1=w5602:sgl[], element #2=w5601:sgl[])  [unwired: 2 in]
                              n2532 = local read "OCgain"() -> (w5609:sgl)
                              n2533 = call "Unscaledtoscaled.vi"("Unscaled Data"=w5602, "Header Information"=w5615) -> ("Array"=w5614:sgl[])  [unwired: 1 in]
                              n2534 = call "Unscaledtoscaled.vi"("Unscaled Data"=w5601, "Header Information"=w5621) -> ("Array"=w5618:sgl[])  [unwired: 1 in]
                              n2535 = Multiply(x=w5614, y=0.1) -> (x*y=w5611:dbl[])
                              n2536 = Divide(x=w5618, y=w5609) -> (x/y=w5610:sgl[])
                              n2537 = Build Array(w5611, w5610) -> (w5613:dbl[][])
                              n2538 = Multiply(x=w5613, y=1000.0) -> (x*y=w5607:dbl[][])
                              "Patch readout" <- w5607
                            }
                            frame #4 {
                              n2539 = case shown="True" w5652 {
                                tunnel: w5651 -> [_ w5664]
                                frame False {
                                }
                                frame True {
                                n2540 = call "patchparameters.vi"("command"="get") -> ("Params out"=w5668:T13)  [unwired: 1 in]
                                n2541 = Unbundle By Name(w5668) -> ("holdon"=w5667:bool, "Vhold (mV)"=w5666:sgl, "CC_icg (pA/mv)"=w5674:sgl, "CC"=w5672:bool, "VC_icg (mV/mV)"=w5673:sgl)
                                n2542 = Select(t=w5674, s=w5672, f=w5673) -> (s? t:f=w5675:sgl)
                                n2543 = To Single Precision Float(number=0.001 ("y")) -> (single precision float=w5676:sgl)
                                n2544 = Compound Arithmetic op=MULTIPLY(w5666, w5675, w5676) -> (w5670:sgl)
                                n2545 = case shown="True" w5667 {
                                tunnel: w5670 -> [_ w5681]
                                tunnel: [0.0 w5681] -> w5665
                                frame False {
                                }
                                frame True {
                                }
                                }
                                n2546 = flat-sequence {
                                tunnel: w5664 -> [w5677]
                                tunnel: w5665 -> [w5679]
                                tunnel: w5664 -> [w5678]
                                frame #0 {
                                n2547 = call "prepAI_sealtest.vi"("samples per channel"=w5677) -> ()  [unwired: 2 in]
                                }
                                frame #1 {
                                n2548 = call "prepAO_sealtest.vi"("Vhold"=w5679, "samples per channel"=w5678) -> ()  [unwired: 1 in]
                                }
                                }
                                }
                              }
                              n2549 = call "sealtestwfparams.vi"("command"="get") -> ("Params out"=w5657:T22)  [unwired: 6 in]
                              n2550 = Unbundle By Name(w5657) -> ("AO parameters"=w5658:T23)
                              n2551 = Index Array(array=w5658, index=0) -> (element=w5660:T24)
                              n2552 = Unbundle By Name(w5660) -> ("Cycles"=w5655:dbl, "Start amplitude (V)"=w5654:dbl, "Sampling frequency (Hz)"=w5653:dbl)
                              n2553 = local read "fitpoints"() -> (w5661:dbl)
                              n2554 = script code="V=data(1,:);\nI=data(2,:);\ntres=mean(V);\nspc=(nsamp./ncyc);\nV=V(spc+1:end-spc);\nI=I(spc+1:end-spc);\ndV=mean(V(V>tres))-mean(V(V<tres))\nIcyc=reshape(I,[spc ncyc-2]);\nIcyc=Icyc';\nIcyc=mean(Icyc,1);\ndIss=mean(Icyc(floor(spc*0.15):floor(spc/2)-2))-mean(Icyc(spc*0.65:spc-2))\nRm=dV*1e3/dIss;\n[maxi,ind]=max(Icyc);\nIfit=Icyc(ind+1:ind+1+points-1)-0.5*(mean(Icyc(floor(spc*0.15):floor(spc/2)-2))+mean(Icyc(spc*0.65:spc-2)))\nt=(3:points-1+3)./srate*1000;\nt=t';\nIfit=Ifit';\nc=fit(t,Ifit, 'exp1');\ncoeffs=coeffvalues(c);\nIa=coeffs(1);\nRa=dV*1e3./Ia/2;\ntau=-1./coeffs(2);\ncap=tau/Ra*1000;"("data"=w5663, "nsamp"=w5651, "ncyc"=w5655, "maxV"=w5654, "points"=w5661, "srate"=w5653) -> ("cap"=w5650:dbl, "Ra"=w5649:dbl, "Icyc"=w5648:dbl[], "Rm"=w5647:dbl)  [unwired: 1 in, 1 out]
                              n2555 = local read "set as Rp?"() -> (w5662:bool)
                              n2556 = local write "Cmembrane"(w5650) -> ()
                              n2557 = local write "Rmembrane (MOhm)"(w5647) -> ()
                              n2558 = local write "Racces (MOhm)"(w5649) -> ()
                              n2559 = case shown="True" w5662 {
                                tunnel: w5647 -> [_ w5682]
                                frame False {
                                }
                                frame True {
                                n2560 = local write "Rpipette (MOhm)"(w5682) -> ()
                                }
                              }
                              n2561 = local write "Ifit"(w5648) -> ()
                            }
                            frame #5 {
                              n2562 = local read "set as Rp?"() -> (w5684:bool)
                              n2563 = case shown="True" w5683 {
                                frame False {
                                }
                                frame True {
                                n2564 = stacked-sequence {
                                frame #0 {
                                n2565 = call "tempconfigAO.vi"("command"="get") -> ("Temp Config out"=w5691:T25)  [unwired: 1 in]
                                n2566 = Unbundle By Name(w5691) -> ("AO"=w5690:refnum<k21>[], "E_AO"=w5689:errorcluster[])
                                n2567 = for {
                                tunnel: w5690 -> [w5698] mode=indexing
                                tunnel: w5689 -> [w5697] mode=indexing
                                tunnel: [w5696] -> w5687 mode=indexing
                                tunnel: [w5695] -> w5686 mode=indexing
                                n2568 = call <vilib>:"DAQmx Start Task.vi"("task/channels in"=w5698, "error in"=w5697) -> ("task out"=w5696:refnum<k21>, "error out"=w5695:errorcluster)  [unwired: 12 in]
                                }
                                n2569 = call "tempconfigAO.vi"("command"="get") -> ("Temp Config out"=w5688:T25)  [unwired: 1 in]
                                n2570 = Bundle By Name(cluster=w5688, "AO"=w5687, "E_AO"=w5686) -> (w5685:T25)
                                n2571 = call "tempconfigAO.vi"("Temp Config in"=w5685, "command"="set") -> ()  [unwired: 1 out]
                                }
                                frame #1 {
                                n2572 = call "tempconfigAI.vi"("command"="get") -> ("Temp Config out"=w5700:T26)  [unwired: 1 in]
                                n2573 = Unbundle By Name(w5700) -> ("AI"=w5705:refnum<k21>, "E_AI"=w5706:errorcluster)
                                n2574 = call <vilib>:"DAQmx Start Task.vi"("task/channels in"=w5705, "error in"=w5706) -> ("task out"=w5707:refnum<k21>, "error out"=w5708:errorcluster)  [unwired: 12 in]
                                n2575 = call "tempconfigAI.vi"("command"="get") -> ("Temp Config out"=w5702:T26)  [unwired: 1 in]
                                n2576 = Bundle By Name(cluster=w5702, "AI"=w5707, "E_AI"=w5708) -> (w5704:T26)
                                n2577 = call "tempconfigAI.vi"("Temp Config in"=w5704, "command"="set") -> ()  [unwired: 1 out]
                                }
                                }
                                }
                              }
                              n2578 = case shown="True" w5684 {
